vi "Trim Data (by ref).vi"(0 "length":u32=20, 1 "Boolean":bool, 11 "Pretrigger Size":i32, 12 "Array":sgl[][](array[numeric])) -> (3 "Data Out":sgl[][](array[numeric]), 13 "Current Size":dbl, 14 "Elements Deleted":dbl)   [LabVIEW 2023]
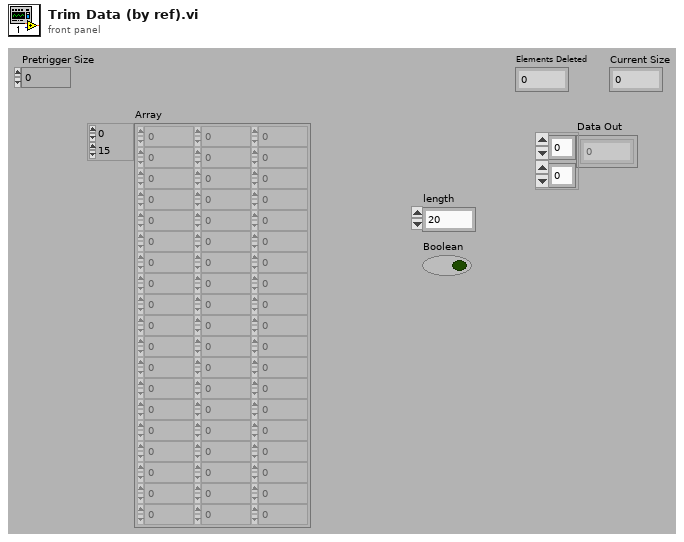
[diagram p1: front panel]
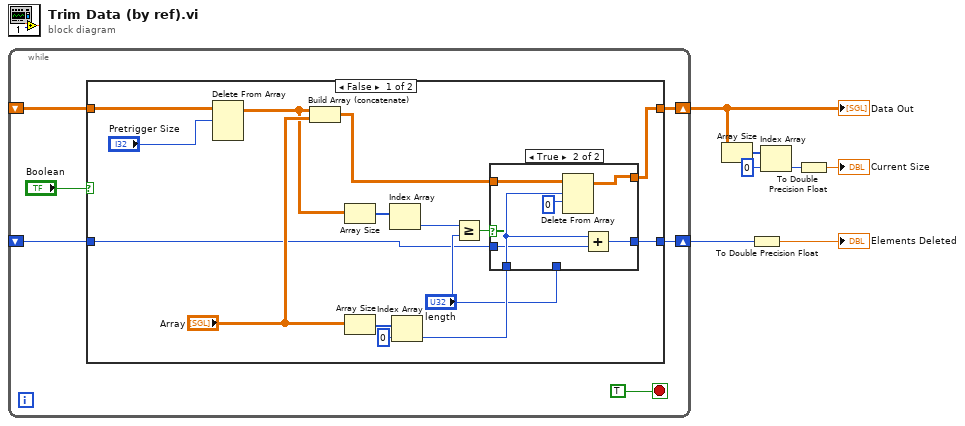
[diagram p0: block diagram]
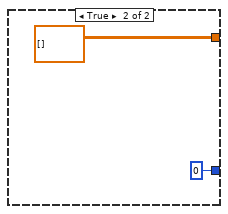
[diagram p3: hidden frame]
diagram:
  n1 = while {
    shift-right: [w12] -> w3
    shift-left: _ -> [w11]
    shift-right: [w9] -> w7
    shift-left: _ -> [w8]
    stop <- TRUE stop-if-true
    n2 = case shown="False" "Boolean" {
      tunnel: [w28 sgl[][] []] -> w12
      tunnel: w11 -> [w16 _]
      tunnel: [w18 0] -> w9
      tunnel: w8 -> [w17 _]
      frame False {
        n3 = Delete From Array(array=w16, length="Pretrigger Size") -> (array with subset deleted=w15:sgl[][])  [unwired: 2 in, 1 out]
        n4 = Build Array (concatenate)(w15, "Array") -> (w27:sgl[][])
        n5 = Array Size(array=w15) -> (size(s)=w26:i32[])
        n6 = Array Size(array="Array") -> (size(s)=w25:i32[])
        n7 = Index Array(array=w26) -> (element=w22:i32)  [unwired: 1 in]
        n8 = Index Array(array=w25, index=0) -> (element=w21:i32)
        n9 = Greater Or Equal?(x=w22, y="length") -> (x >= y?=w24:bool)
        n10 = case shown="True" w24 {
          tunnel: w27 -> [w30 w36]
          tunnel: [w30 w35] -> w28
          tunnel: w21 -> [_ w33]
          tunnel: "length" -> [_ _]
          tunnel: [w29 w32] -> w18
          tunnel: w17 -> [w29 w31]
          frame False {
          }
          frame True {
            n11 = Delete From Array(array=w36, length=w33, index (row)=0) -> (array with subset deleted=w35:sgl[][])  [unwired: 1 in, 1 out]
            n12 = Add(x=w33, y=w31) -> (x+y=w32:i32)
          }
        }
      }
      frame True {
      }
    }
  }
  "Data Out" <- w3
  n13 = Array Size(array=w3) -> (size(s)=w6:i32[])
  n14 = To Double Precision Float(number=w7) -> (double precision float=→"Elements Deleted":dbl)
  n15 = Index Array(array=w6, index=0) -> (element=w4:i32)
  n16 = To Double Precision Float(number=w4) -> (double precision float=→"Current Size":dbl)
